vi "XMLAppendPosToConfig.vi"(8 "error in (no error)":errorcluster, 9 "ItemNames":string[][](array[string]), 10 "Only Position?":bool, 11 "selected path":path) -> (0 "error out":errorcluster, 3 "XML":string)   [LabVIEW 2018]
uses:
  <vilib>/xml/Load XML File.vi
  <vilib>/xml/NI_XML.lvlib
  <resource>/objmgr/DOMUserDefRef.rc
panel:
  out "XML 2":string
  out "parse errors":string
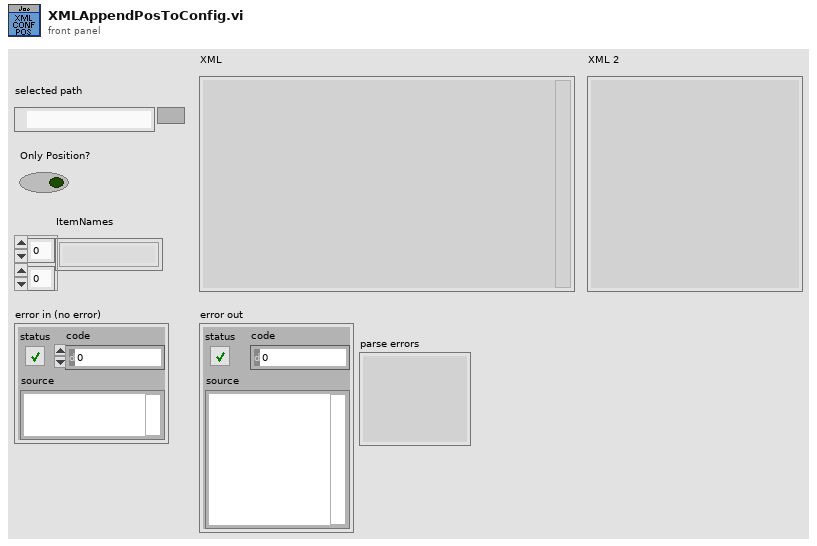
[diagram p1: front panel]
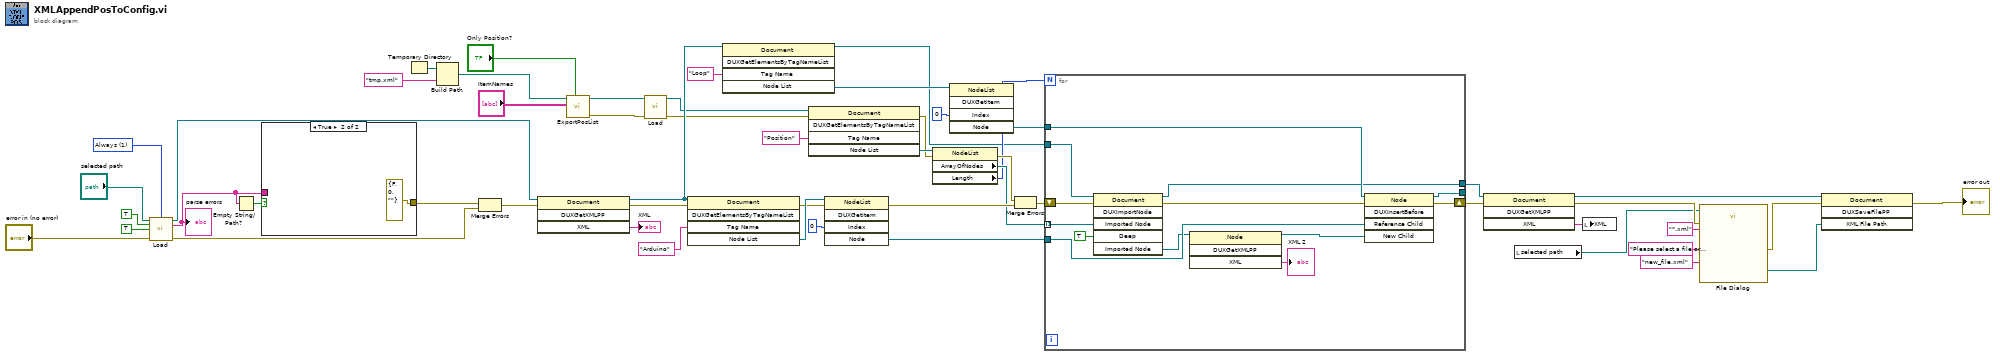
[diagram p0: block diagram]
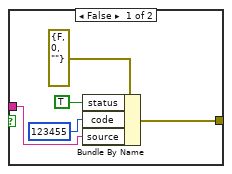
[diagram p2: hidden frame]
diagram:
  w45 = 1 items=["Never", "Always", "Auto"] ("validate on load (Auto)")
  n1 = call-poly <vilib>:"Load.vi"("path to XML document"="selected path", "validate on load (Auto)"=w45, "process namespaces (False)"=TRUE, "process schema (False)"=TRUE, "error in (no error)"="error in (no error)") -> ("DOM document out"=w42:refnum<k20>, "parse errors"=w34:string, "error out"=w33:errorcluster)  [unwired: 8 in]
  "parse errors" <- w34
  n2 = Empty String/Path?(string/path=w34) -> (empty?=w35:bool)
  n3 = case shown="True" w35 {
    tunnel: w34 -> [w55 _]
    tunnel: [w54 errorcluster {"status"=FALSE, "code"=0, "source"=""} ("error in")] -> w32
    frame False {
      n4 = Bundle By Name(cluster=errorcluster {"status"=FALSE, "code"=0, "source"=""} ("error in"), "status"=TRUE, "code"=123455, "source"=w55) -> (w54:errorcluster)
    }
    frame True {
    }
  }
  n5 = Temporary Directory() -> (w38:path)
  n6 = Build Path(base path=w38, name or relative path="tmp.xml") -> (appended path=w39:path)
  n7 = Merge Errors(w32, w33) -> (w36:errorcluster)
  n8 = invoke class="Document" method="DUXGetXMLPP"(reference=w42, error in=w36) -> (reference out=w19:refnum<k20>, error out=w46:errorcluster, "XML"=→"XML":string)  [unwired: 2 in, 1 out]
  n9 = call "ExportPosList.vi"("XML File Path"=w39, "Array"="ItemNames", "Only Pos"="Only Position?") -> ("XML File Path Out"=w31:path, "error out"=w29:errorcluster)  [unwired: 6 in]
  n10 = call-poly <vilib>:"Load.vi"("path to XML document"=w31, "error in (no error)"=w29) -> ("DOM document out"=w15:refnum<k20>, "error out"=w14:errorcluster)  [unwired: 11 in, 1 out]
  n11 = invoke class="Document" method="DUXGetElementsByTagNameList"(reference=w19, error in=w46, "Tag Name"="Arduino") -> (error out=w49:errorcluster, "Node List"=w50:refnum<k20>)  [unwired: 2 in, 3 out]
  n12 = invoke class="Document" method="DUXGetElementsByTagNameList"(reference=w19, "Tag Name"="Loop") -> (reference out=w13:refnum<k20>, "Node List"=w17:refnum<k20>)  [unwired: 3 in, 3 out]
  n13 = invoke class="Document" method="DUXGetElementsByTagNameList"(reference=w15, error in=w14, "Tag Name"="Position") -> (error out=w25:errorcluster, "Node List"=w26:refnum<k20>)  [unwired: 2 in, 3 out]
  n14 = invoke class="NodeList" method="DUXGetItem"(reference=w50, error in=w49, "Index"=0) -> (error out=w27:errorcluster, "Node"=w21:refnum<k20>)  [unwired: 2 in, 3 out]
  n15 = property class="NodeList"(reference=w26, error in=w25) -> (error out=w24:errorcluster, "ArrayOfNodes"=w23:refnum<k20>[], "Length"=w22:i32)  [unwired: 1 out]
  n16 = invoke class="NodeList" method="DUXGetItem"(reference=w17, "Index"=0) -> ("Node"=w16:refnum<k20>)  [unwired: 3 in, 4 out]
  n17 = Merge Errors(w24, w27) -> (w28:errorcluster)
  n18 = for {
    N: w22 -> [_]
    tunnel: w23 -> [w67] mode=indexing
    tunnel: w16 -> [w72]
    tunnel: w21 -> [w69]
    shift-right: [w71] -> w10
    shift-left: w28 -> [w63]
    tunnel: [w70] -> _
    tunnel: w13 -> [w68]
    tunnel: [w64] -> w12
    n19 = invoke class="Document" method="DUXImportNode"(reference=w68, error in=w63, "Imported Node"=w67, "Deep"=TRUE) -> (reference out=w64:refnum<k20>, error out=w62:errorcluster, "Imported Node"=w66:refnum<k20>)  [unwired: 2 in, 3 out]
    n20 = invoke class="Node" method="DUXGetXMLPP"(reference=w66) -> (reference out=w61:refnum<k20>, "XML"=→"XML 2":string)  [unwired: 3 in, 2 out]
    n21 = invoke class="Node" method="DUXInsertBefore"(reference=w72, error in=w62, "Reference Child"=w69, "New Child"=w61) -> (reference out=w70:refnum<k20>, error out=w71:errorcluster)  [unwired: 1 in, 3 out]
  }
  n22 = invoke class="Document" method="DUXGetXMLPP"(reference=w12, error in=w10) -> (reference out=w9:refnum<k20>, error out=w6:errorcluster, "XML"=w11:string)  [unwired: 2 in, 1 out]
  n23 = local read "selected path"() -> (w1:path)
  n24 = local write "XML"(w11) -> ()
  n25 = call "File Dialog"("start path"=w1, "prompt"="Please select a file or specify a new filename to save the configuration", "default name"="new_file.xml", "error in"=w6, "pattern (all files)"="*.xml") -> ("selected path"=w7:path, "error out"=w5:errorcluster)  [unwired: 7 in, 2 out]
  n26 = invoke class="Document" method="DUXSaveFilePP"(reference=w9, error in=w5, "XML File Path"=w7) -> (error out=→"error out":errorcluster)  [unwired: 1 in, 3 out]
